vi "us_to_ms_EXT.vi"(4 "time in":ext caption="time in [µs]" format="%#.6f") -> (1 "time out":ext caption="time out [ms]" format="%#.6f")   [LabVIEW 2017, in "GPTiming.lvlib"]
doc: "Divides <B>time in</B> by 1,000 to convert it from microseconds to milliseconds.\n\nEven though its functionality is really simple this function is valuable as it documents your code much better than a raw division by 1,000.\n\nThis VI is inlined.\n\nSteen Schmidt\nGPower\n9/12 2013"
uses:
  GPTiming.lvlib
panel:
  # "Copyright © 2013\nGPower\nSee enclosed license file for terms and conditions"
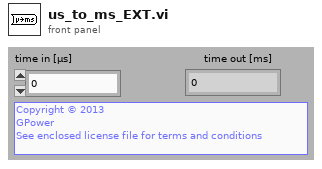
[diagram p1: front panel]
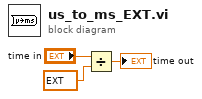
[diagram p0: block diagram]
diagram:
  n1 = Divide(x="time in", y=ext 1000.0) -> (x/y=→"time out":ext)
